vi "Query.vi"(8 "error in":errorcluster, 10 "Query":string, 11 "89XX in":refnum<class "89XX.lvclass">) -> (0 "error out":errorcluster, 2 "Response":string, 3 "89XX out":refnum<class "89XX.lvclass">)   [LabVIEW 2019, in "89XX.lvlib" / "89XX.lvclass"]
uses:
  Library/89XX.lvclass
  Library/89XX.lvclass/89XX.ctl
  <instrlib>/Keysight N8900 Series/Keysight N8900 Series.lvlib
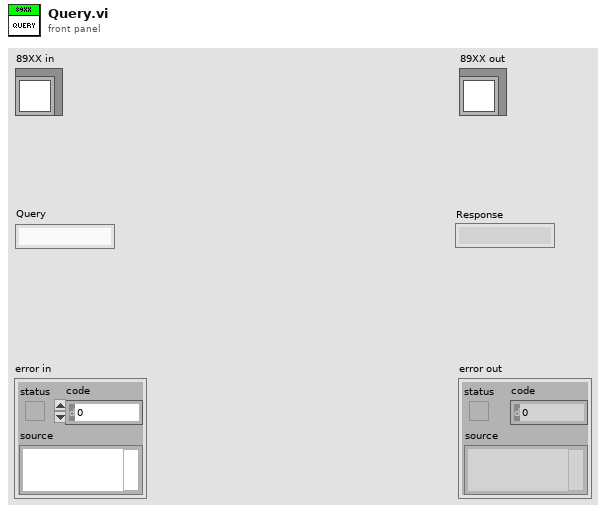
[diagram p1: front panel]
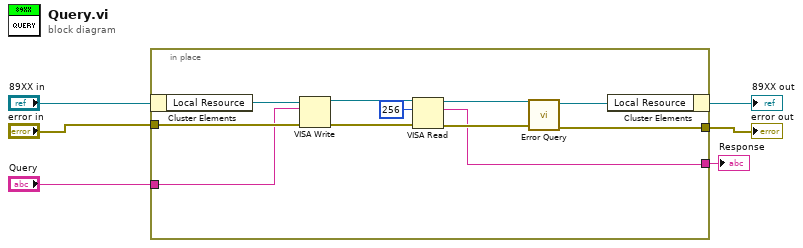
[diagram p0: block diagram]
diagram:
  n1 = in-place {
    in-place-border: [w16] -> w4
    in-place-border: "error in" -> [w10]
    in-place-border: [w9] -> w2
    in-place-border: "Query" -> [w8]
    n2 = in-place-cluster #1("89XX in") -> ("Local Resource"=w13:refnum<visa-resource-name>)
    n3 = VISA Write(VISA resource name=w13, write buffer=w8, error in (no error)=w10) -> (VISA resource name out=w15:refnum<visa-resource-name>, error out=w12:errorcluster)  [unwired: 1 out]
    n4 = VISA Read(VISA resource name=w15, byte count=u32 256, error in (no error)=w12) -> (VISA resource name out=w14:refnum<visa-resource-name>, read buffer=w9:string, error out=w11:errorcluster)  [unwired: 1 out]
    n5 = call <instrlib>:"Error Query.vi"("error in (no error)"=w11, "VISA resource name"=w14) -> ("error out"=w16:errorcluster, "VISA resource name out"=w17:refnum<visa-resource-name>)  [unwired: 6 in, 2 out]
    n6 = in-place-cluster #1("Local Resource"=w17) -> (→"89XX out":refnum<class "89XX.lvclass">)
  }
  "error out" <- w4
  "Response" <- w2
